vi "Oriental_step_motor_PKP214.vi"(6 "tau_Threshold":fxp<+,12,12>, 8 "dtaumr":fxp<+/-,25,15>, 10 "omega":fxp<+/-,20,9>, 11 "taumr":fxp<+/-,21,11>) -> (1 "vq_F":fxp<+/-,20,5> format="%.57g", 3 "vd_F":fxp<+/-,20,5>)   [LabVIEW 2014]
uses:
  <vilib>/rvi/FXPMathLib/FxpMul/XNode/nifxpmath_Multiplier.xnode
  <vilib>/rvi/FXPMathLib/FxpAdd/XNode/nifxpmath_Add.xnode
  <vilib>/rvi/FXPMathLib/sim/FxpSim.dll
panel:
  out "Lmdtau_mr/Km":fxp<+/-,30,15>
  out "-RKm/NrL":fxp<+/-,18,3>=-1.9615478515625
  out "tauR/Km":fxp<+/-,30,15>
  out "Kmw":fxp<+/-,25,10> format="%.50g"
  out "-NrLwtau/Km":fxp<+/-,28,9> format="%.54g"
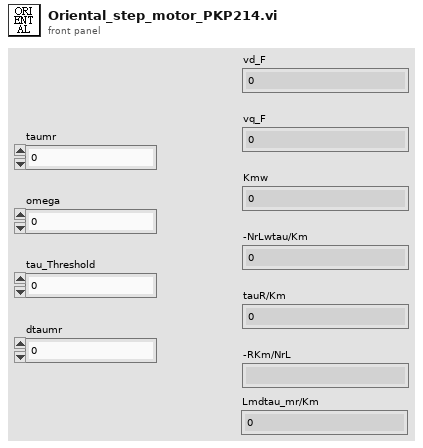
[diagram p1: front panel]
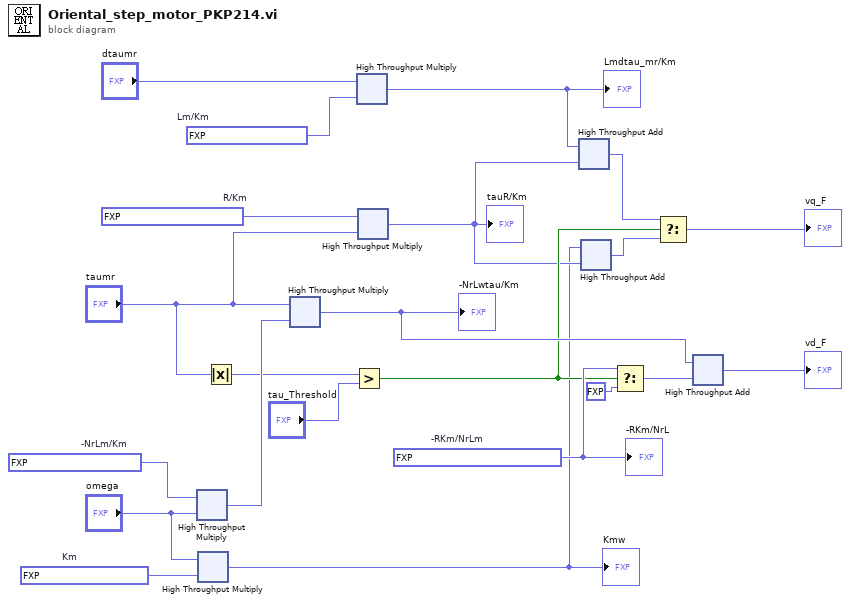
[diagram p0: block diagram]
diagram:
  w17 = fxp<+,23,7> 0.095123291015625  # Lm/Km
  w15 = fxp<+/-,20,4> -4.7561187744140625  # -NrLm/Km
  w13 = fxp<+/-,25,4> -1.2902369499206543  # -RKm/NrLm
  w19 = fxp<+,24,8> 183.17970275878906  # R/Km
  w12 = fxp<+,14,-2> 0.0334930419921875  # Km
  n1 = xnode ("High Throughput Multiply")("x"=w15, "y"="omega") -> ("x*y"=w14:fxp<+/-,28,9>)
  n2 = xnode ("High Throughput Multiply")("x"="omega", "y"=w12) -> ("x*y"=w3:fxp<+/-,22,7>)
  "Kmw" <- w3
  n3 = Absolute Value(x="taumr") -> (abs(x)=w10:fxp<+,21,11>)
  n4 = xnode ("High Throughput Multiply")("x"="taumr", "y"=w14) -> ("x*y"=w8:fxp<+/-,28,9>)
  "-NrLwtau/Km" <- w8
  n5 = Greater?(x=w10, y="tau_Threshold") -> (0:w6:bool)
  n6 = xnode ("High Throughput Multiply")("x"="dtaumr", "y"=w17) -> ("x*y"=w16:fxp<+/-,20,5>)
  "Lmdtau_mr/Km" <- w16
  n7 = xnode ("High Throughput Multiply")("x"=w19, "y"="taumr") -> ("x*y"=w4:fxp<+/-,20,5>)
  "tauR/Km" <- w4
  n8 = xnode ("High Throughput Add")("x"=w16, "y"=w4) -> ("x+y"=w18:fxp<+/-,20,5>)
  n9 = xnode ("High Throughput Add")("x"=w3, "y"=w4) -> ("x+y"=w5:fxp<+/-,20,5>)
  n10 = Select(t=w13, s=w6, f=fxp<+/-,18,3> 0.0) -> (s? t:f=w7:fxp<+/-,25,4>)
  n11 = Select(t=w18, s=w6, f=w5) -> (s? t:f=→"vq_F":fxp<+/-,20,5>)
  n12 = xnode ("High Throughput Add")("x"=w8, "y"=w7) -> ("x+y"=→"vd_F":fxp<+/-,20,5>)
  "-RKm/NrL" <- w13
